vi "case.vi"() -> ()   [LabVIEW 2013]
panel:
  in  "Boolean 2":bool
  out "Boolean 3":bool
  out "Numeric  while false":dbl
  out "Numeric   for true":dbl
  in  "Boolean":bool
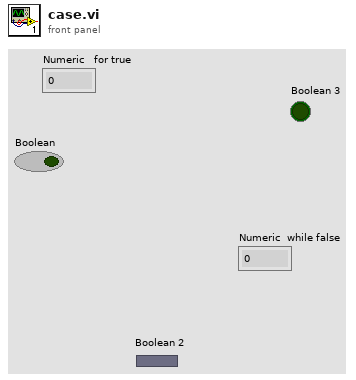
[diagram p1: front panel]
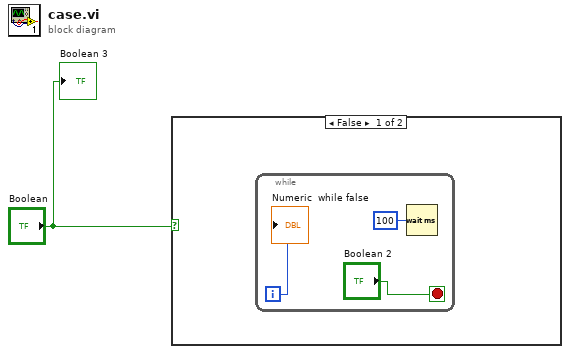
[diagram p0: block diagram]
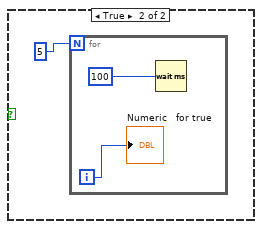
[diagram p2: hidden frame]
diagram:
  n1 = case shown="False" "Boolean" {
    frame False {
      n2 = while {
        i -> [w3]
        stop <- "Boolean 2" stop-if-true
        n3 = Wait (ms)(milliseconds to wait=u32 100) -> ()  [unwired: 1 out]
        "Numeric  while false" <- w3
      }
    }
    frame True {
      n4 = for {
        N: 5 -> [_]
        i -> [w7]
        n5 = Wait (ms)(milliseconds to wait=u32 100) -> ()  [unwired: 1 out]
        "Numeric   for true" <- w7
      }
    }
  }
  "Boolean 3" <- "Boolean"
